vi "Memory.Pointer.Read.Safe.1D.I64.vi"(8 "error in (no error)":errorcluster, 9 "count":u64 format="%d elements", 10 "buffer in":i64[](array[numeric]), 11 "pointer in":refnum<class "Memory.Pointer.lvclass">) -> (0 "error out":errorcluster, 1 "count out":u64 format="%d elements", 2 "buffer out":i64[](array[numeric]), 3 "pointer out":refnum<class "Memory.Pointer.lvclass">)   [LabVIEW 2016, in "Memory Manager.lvlib" / "Memory.Pointer.lvclass"]
doc: "Reads <b>count</b> elements from the address specified by <b>pointer</b> into the provided <b>buffer</b>.\n\n<b>Note:</b> This VI is <b>safe</b>.\n\nSafe means that this function evaluates the size parameter of <b>pointer</b> to ensure that is inbounds of allocated memory before peforming a memory read/write. Reading/writing more data to a pointer than it has allocated can corrupt or crash LabVIEW."
uses:
  Memory.Pointer.lvclass
  Memory.Pointer.lvclass/Memory.Pointer.ctl
  Accessors/Get Address.vi
  Memory.Pointer.Errors.vi
  Memory.Pointer.Errors.Buffer Underflow.vi
  Memory.Pointer.Parameter Check.Size.vi
  Memory.Pointer.Errors.Create Error.vi
  Submodules/Static Error Handling/Source/Library/VIs/Static Error Handling.Source Buffer.Write.String.vi
  Submodules/Static Error Handling/Source/Library/VIs/Static Error Handling.Source Buffer.Write.Numeric.Scalar.Base10.vi
  Submodules/Static Error Handling/Source/Library/VIs/Static Error Handling.Source Buffer.Write.Numeric.Scalar.Base10 (U64).vi
  Memory.Pointer.Errors.Out of Bounds.vi
  Accessors/Get Size.vi
  Submodules/Static Error Handling/Source/Library/VIs/Static Error Handling.Error Cluster Constant.vi
  Submodules/Static Error Handling/Source/Library/VIs/Static Error Handling.Error Cluster Constant (256B).vi
  Submodules/Static Error Handling/Source/Library/VIs/Static Error Handling.Parameters.Status.Set.vi
  Submodules/Static Error Handling/Source/Library/VIs/Static Error Handling.Parameters.Code.Set.vi
  Submodules/Static Error Handling/Source/Library/VIs/Static Error Handling.Parameters.VI Source.Set.vi
  Constants/Memory.Constants.vi
  Constants/Memory.Constants.Library Name.vi
  Memory.Pointer.Errors.Get Info.vi
  Memory.Pointer.Errors.Write Pointer Size.vi
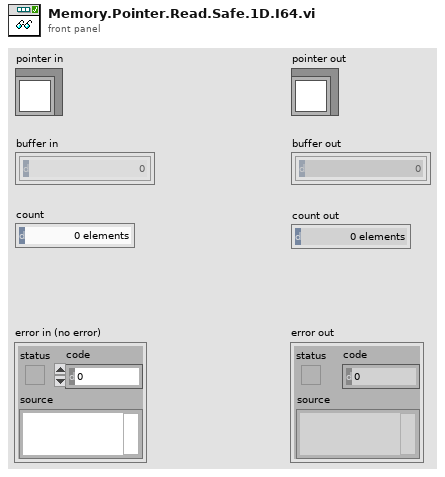
[diagram p1: front panel]
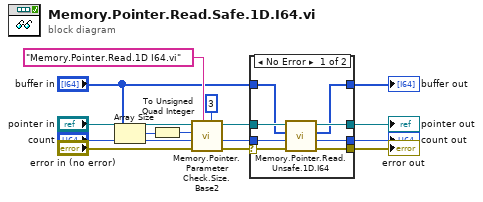
[diagram p0: block diagram]
diagram:
  n1 = Array Size(array="buffer in") -> (size(s)=w15:i32)
  n2 = To Unsigned Quad Integer(1:w15) -> (0:w14:u64)
  n3 = call "Memory.Pointer.Parameter Check.Size.Base2.vi"("power of 2"=i16 3, "source vi name"="Memory.Pointer.Read.1D I64.vi", "error in (no error)"="error in (no error)", "transfer count"="count", "buffer element count"=w14, "Pointer in"="pointer in") -> ("error out"=w13:errorcluster, "transfer count out"=w11:u64, "Pointer out"=w12:refnum<class "Memory.Pointer.lvclass">)  [unwired: 2 in, 1 out]
  n4 = case shown="No Error" w13 {
    selector: w13 -> [w23 w26]
    tunnel: w12 -> [w21 w25]
    tunnel: w11 -> [w22 w27]
    tunnel: "buffer in" -> [w17 w24]
    tunnel: [w20 w26] -> w4
    tunnel: [w19 w25] -> w1
    tunnel: [w18 w27] -> w3
    tunnel: [w16 w24] -> w7
    frame No Error {
      n5 = call "Memory.Pointer.Read.Unsafe.1D.I64.vi"("error in (no error)"=w23, "count"=w22, "buffer in"=w17, "pointer in"=w21) -> ("error out"=w20:errorcluster, "count out"=w18:u64, "buffer out"=w16:i64[], "pointer out"=w19:refnum<class "Memory.Pointer.lvclass">)  [unwired: 4 in]
    }
    frame Error {
    }
  }
  "error out" <- w4
  "pointer out" <- w1
  "buffer out" <- w7
  "count out" <- w3
